vi "FTW-Actor-AsyncLaunch.vi"(0 "FTW Actor Instance Type":refnum<class "FTW-ActorInstance.lvclass">, 7 "Actor Instance Configuration":string, 11 "error in":errorcluster) -> (15 "error out":errorcluster)   [LabVIEW 2015, in "FTW-ActorInstance.lvclass"]
doc: "This VI exists to call the dynamic dispatch actor since dynamic dispatch VIs cannot be called by reference"
uses:
  FTW-ActorInstance.lvclass
panel:
  # "Inputs"
  # "Outputs"
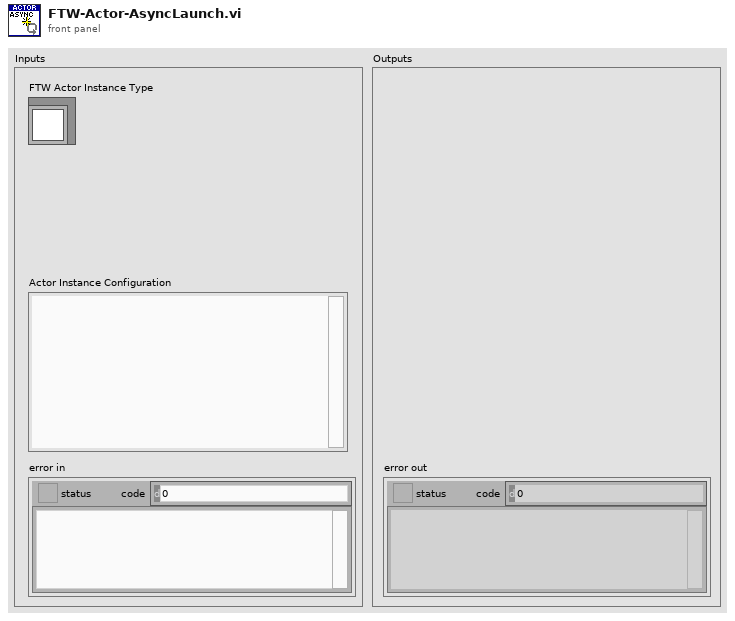
[diagram p1: front panel]
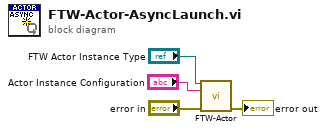
[diagram p0: block diagram]
diagram:
  n1 = call-dynamic "FTW-Actor.vi"("FTW Actor Instance"="FTW Actor Instance Type", "FTW Actor Instance Configuration"="Actor Instance Configuration", "ErrorIn"="error in") -> ("Error"=→"error out":errorcluster)  [unwired: 12 in]
